vi "create_arb_waveform.vi"(0 "Waveform Parameters":T1={"Function"=enum."Exponential", "Initial"=0.0, "Final"=0.0, "Degree"=1.0, "Nickname"="", "Conversion"=enum."B Field Grad (G/cm)", "Constant"=0.0} {"Degree" min=1.0}, 1 "Sample rate":dbl, 2 "Time":dbl) -> (3 "Samples to Write":dbl, 4 "dt":dbl, 5 "Tau (exponential)":dbl, 6 "output waveform":waveform(dbl)(graph))   [LabVIEW 2016]
uses:
  6733_Red_MOT/6733_waveform_item.ctl
  6733_Red_MOT/Neutral_voltage_conversion_control.ctl
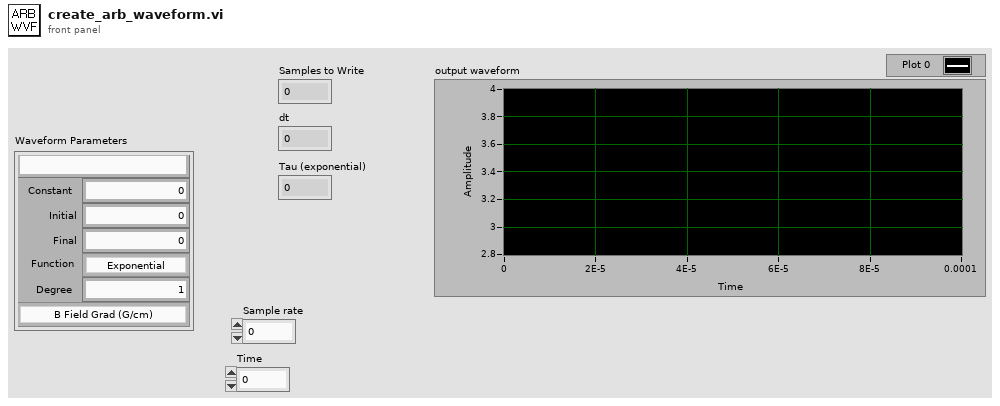
[diagram p1: front panel]
types:
  T1 = typedef "6733_waveform_item.ctl" = cluster{"Function":enum16{"Polynomial", "Exponential", "Constant", "Tanh"}, "Initial":dbl, "Final":dbl, "Degree":dbl, "Nickname":string, "Conversion":T2, "Constant":dbl}
  T2 = typedef "Neutral_voltage_conversion_control.ctl" = enum16{"Volts", "B Field Grad (G/cm)", "Red Boson Cntr Freq (MHz)", "Red Boson Dither Amp (kHz)", "Red Boson Power (mW)", "Red 87 Trap Cntr Freq (MHz)", "Red 87 Trap Dither Amp (kHz)", "Red 87 Trap Power (mW)", "Red 87 Stir Cntr Freq (MHz)", "Red 87 Stir Dither Amp (kHz)", "Red 87 Stir Power (mW)", "ODT Sheet Trap Power (W)", "ODT Loading Trap Power (W)"}
  T3 = cluster{"Waveform Parameters":T1, "Time":dbl, "Sample rate":dbl}
  T4 = enum16{"Polynomial", "Exponential", "Constant", "Tanh"}
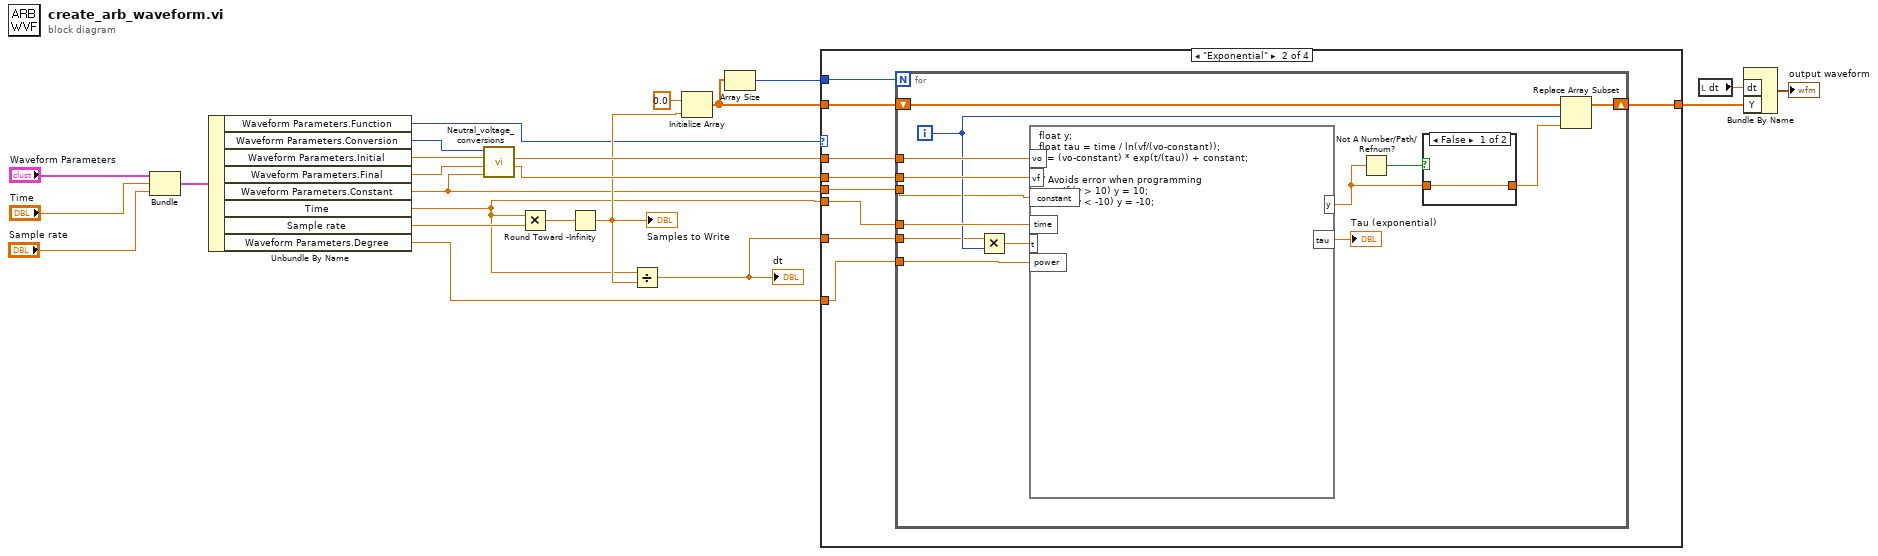
[diagram p0: block diagram]
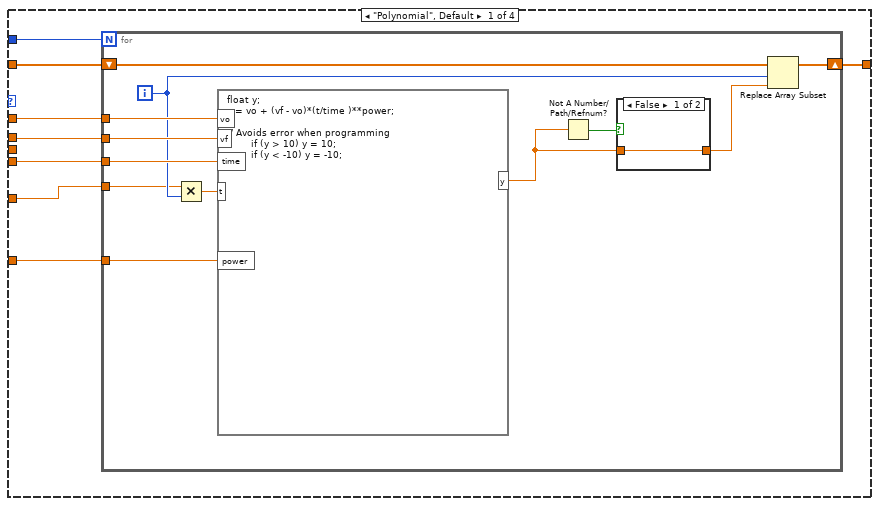
[diagram p2: hidden frame]
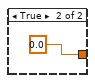
[diagram p3: hidden frame]
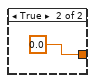
[diagram p4: hidden frame]
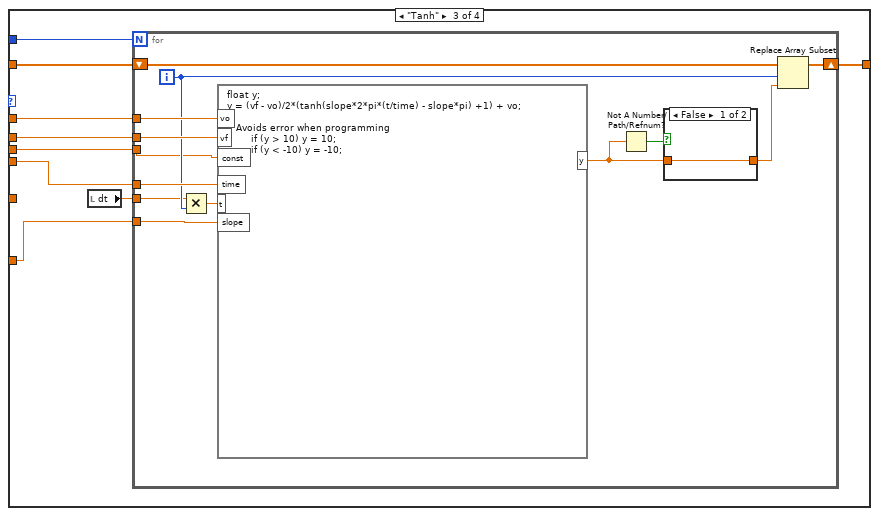
[diagram p5: hidden frame]
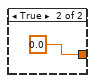
[diagram p6: hidden frame]
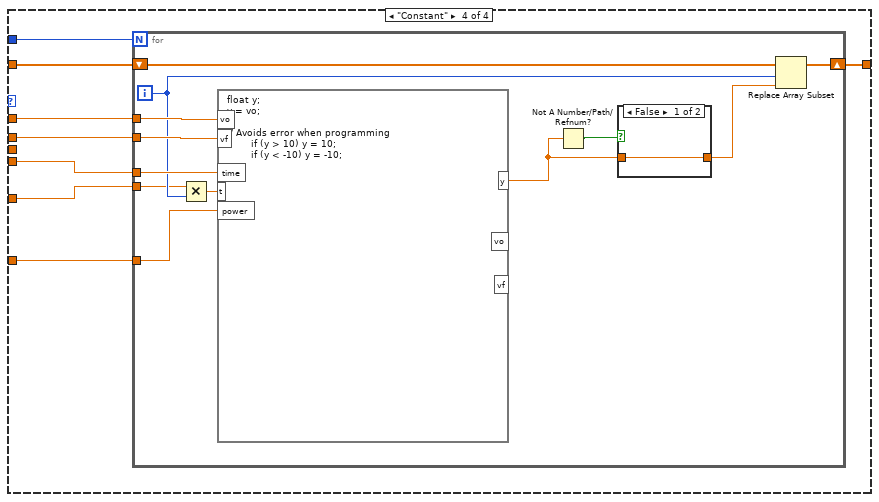
[diagram p7: hidden frame]
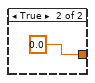
[diagram p8: hidden frame]
diagram:
  n1 = Bundle("Waveform Parameters"="Waveform Parameters", "Time"="Time", "Sample rate"="Sample rate") -> (w13:T3)  [unwired: 1 in]
  n2 = Unbundle By Name(w13) -> ("Waveform Parameters.Function"=w7:T4, "Waveform Parameters.Conversion"=w12:T2, "Waveform Parameters.Initial"=w6:dbl, "Waveform Parameters.Final"=w5:dbl, "Waveform Parameters.Constant"=w2:dbl, "Time"=w1:dbl, "Sample rate"=w9:dbl, "Waveform Parameters.Degree"=w4:dbl)
  n3 = call "Neutral_voltage_conversions.vi"("Constant"=w2, "Final Value"=w5, "Initial value"=w6, "Conversion"=w12) -> ("Final Voltage"=w10:dbl, "Initial voltage"=w11:dbl)  [unwired: 6 in]
  n4 = Multiply(x=w1, y=w9) -> (x*y=w17:dbl)
  n5 = Round Toward -Infinity(1:w17) -> (0:w8:dbl)
  "Samples to Write" <- w8
  n6 = Divide(x=w1, y=w8) -> (x/y=w3:dbl)
  "dt" <- w3
  n7 = Initialize Array(0.0 ("element"), w8) -> (w19:dbl[])
  n8 = Array Size(array=w19) -> (size(s)=w18:i32)
  n9 = case shown="\"Exponential\"" w7 {
    tunnel: w19 -> [w31 w54 w79 w102]
    tunnel: [w30 w53 w78 w101] -> w22
    tunnel: w11 -> [w29 w52 w77 w100]
    tunnel: w10 -> [w28 w51 w76 w99]
    tunnel: w1 -> [w27 w50 w75 w98]
    tunnel: w18 -> [w26 w49 w73 w97]
    tunnel: w4 -> [w25 w48 w72 w96]
    tunnel: w3 -> [w24 w46 _ w95]
    tunnel: w2 -> [_ w47 w71 _]
    frame "Polynomial", Default {
      n10 = for {
        N: w26 -> [_]
        shift-right: [w42] -> w30
        shift-left: w31 -> [w43]
        tunnel: w29 -> [w41]
        tunnel: w28 -> [w40]
        tunnel: w27 -> [w39]
        tunnel: w24 -> [w36]
        tunnel: w25 -> [w35]
        i -> [w37]
        n11 = Multiply(x=w36, y=w37) -> (x*y=w38:dbl)
        n12 = formula code="float y;\ny = vo + (vf - vo)*(t/time )**power;\n\n// Avoids error when programming\n        if (y > 10) y = 10;\n        if (y < -10) y = -10;"("vo"=w41, "vf"=w40, "time"=w39, "t"=w38, "power"=w35) -> ("y"=w33:dbl)
        n13 = Not A Number/Path/Refnum?(number/path/refnum=w33) -> (NaN/Path/Refnum?=w32:bool)
        n14 = case shown="False" w32 {
          tunnel: [w44 0.0] -> w34
          tunnel: w33 -> [w44 _]
          frame False {
          }
          frame True {
          }
        }
        n15 = Replace Array Subset(array=w43, new element=w34, index=w37) -> (w42:dbl[])
      }
    }
    frame "Exponential" {
      n16 = for {
        N: w49 -> [_]
        shift-right: [w67] -> w53
        shift-left: w54 -> [w68]
        tunnel: w52 -> [w66]
        tunnel: w51 -> [w65]
        tunnel: w50 -> [w64]
        tunnel: w46 -> [w61]
        tunnel: w48 -> [w59]
        tunnel: w47 -> [w58]
        i -> [w62]
        n17 = Multiply(x=w61, y=w62) -> (x*y=w63:dbl)
        n18 = formula code="float y;\nfloat tau = time / ln(vf/(vo-constant));\ny = (vo-constant) * exp(t/(tau)) + constant;\n\n// Avoids error when programming\n        if (y > 10) y = 10;\n        if (y < -10) y = -10;"("vo"=w66, "vf"=w65, "time"=w64, "t"=w63, "power"=w59, "constant"=w58) -> ("y"=w56:dbl, "tau"=→"Tau (exponential)":dbl)
        n19 = Not A Number/Path/Refnum?(number/path/refnum=w56) -> (NaN/Path/Refnum?=w55:bool)
        n20 = case shown="False" w55 {
          tunnel: [w69 0.0] -> w57
          tunnel: w56 -> [w69 _]
          frame False {
          }
          frame True {
          }
        }
        n21 = Replace Array Subset(array=w68, new element=w57, index=w62) -> (w67:dbl[])
      }
    }
    frame "Tanh" {
      n22 = local read "dt"() -> (w74:dbl)
      n23 = for {
        N: w73 -> [_]
        shift-right: [w91] -> w78
        shift-left: w79 -> [w92]
        tunnel: w77 -> [w90]
        tunnel: w76 -> [w89]
        tunnel: w75 -> [w88]
        tunnel: w74 -> [w85]
        tunnel: w72 -> [w84]
        tunnel: w71 -> [w83]
        i -> [w86]
        n24 = Multiply(x=w85, y=w86) -> (x*y=w87:dbl)
        n25 = formula code="float y;\ny = (vf - vo)/2*(tanh(slope*2*pi*(t/time) - slope*pi) +1) + vo;\n\n// Avoids error when programming\n        if (y > 10) y = 10;\n        if (y < -10) y = -10;"("vo"=w90, "vf"=w89, "time"=w88, "t"=w87, "slope"=w84, "const"=w83) -> ("y"=w81:dbl)
        n26 = Not A Number/Path/Refnum?(number/path/refnum=w81) -> (NaN/Path/Refnum?=w80:bool)
        n27 = case shown="False" w80 {
          tunnel: [w93 0.0] -> w82
          tunnel: w81 -> [w93 _]
          frame False {
          }
          frame True {
          }
        }
        n28 = Replace Array Subset(array=w92, new element=w82, index=w86) -> (w91:dbl[])
      }
    }
    frame "Constant" {
      n29 = for {
        N: w97 -> [_]
        shift-right: [w113] -> w101
        shift-left: w102 -> [w114]
        tunnel: w100 -> [w112]
        tunnel: w99 -> [w111]
        tunnel: w98 -> [w110]
        tunnel: w95 -> [w107]
        tunnel: w96 -> [w106]
        i -> [w108]
        n30 = Multiply(x=w107, y=w108) -> (x*y=w109:dbl)
        n31 = formula code="float y;\ny = vo;\n\n// Avoids error when programming\n        if (y > 10) y = 10;\n        if (y < -10) y = -10;"("vo"=w112, "vf"=w111, "time"=w110, "t"=w109, "power"=w106) -> ("y"=w103:dbl)  [unwired: 2 out]
        n32 = Not A Number/Path/Refnum?(number/path/refnum=w103) -> (NaN/Path/Refnum?=w104:bool)
        n33 = case shown="False" w104 {
          tunnel: [w115 0.0] -> w105
          tunnel: w103 -> [w115 _]
          frame False {
          }
          frame True {
          }
        }
        n34 = Replace Array Subset(array=w114, new element=w105, index=w108) -> (w113:dbl[])
      }
    }
  }
  n35 = local read "dt"() -> (w21:dbl)
  n36 = Bundle By Name("dt"=w21, "Y"=w22) -> (→"output waveform":waveform(dbl))  [unwired: 1 in]
